vi "Suggestion Box Panel.vi"(11 "Suggestion Box":refnum<class "Suggestion Box.lvclass">) -> ()   [LabVIEW 2016, in "Suggestion Box.lvclass"]
doc: "Suggestion Box panel process.\n--------------------\nCopyright (c) 2019 Analog Devices, Inc. All rights reserved.\n\nRedistribution and use in source and binary forms, with or without modification,\nare permitted provided that the following conditions are met:\n - Redistributions of source code must retain the above copyright notice, this\n list of conditions and the following disclaimer.\n - Redistributions in binary form must reproduce the above copyright notice,\n this list of conditions and the following disclaimer in the documentation\n and/or other materials provided with the distribution.\n - Modified versions of the software must be conspicuously marked as such.\n - This software is licensed solely and exclusively for use with\n processors/products manufactured by or for Analog Devices, Inc.\n - This software may not be combined or merged with other code in any manner\n that would cause the software to become subject to terms and conditions\n which differ from those listed here.\n - Neither the name of Analog Devices, Inc. nor the names of its contributors\n may be used to endorse or promote products derived from this software\n without specific prior written permission.\n - The use of this software may or may not infringe the patent rights of one or\n more patent holders. This license does not release you from the requirement\n that you obtain separate licenses from these patent holders to use this\n software.\n\nTHIS SOFTWARE IS PROVIDED BY ANALOG DEVICES, INC. AND CONTRIBUTORS \"AS IS\" AND\nANY EXPRESS OR IMPLIED WARRANTIES, INCLUDING, BUT NOT LIMITED TO,\nNON-INFRINGEMENT, TITLE, MERCHANTABILITY AND FITNESS FOR A PARTICULAR PURPOSE\nARE DISCLAIMED. IN NO EVENT SHALL ANALOG DEVICES, INC. OR CONTRIBUTORS BE LIABLE\nFOR ANY DIRECT, INDIRECT, INCIDENTAL, SPECIAL, EXEMPLARY, PUNITIVE OR\nCONSEQUENTIAL DAMAGES (INCLUDING, BUT NOT LIMITED TO, DAMAGES ARISING OUT OF\nCLAIMS OF INTELLECTUAL PROPERTY RIGHTS INFRINGEMENT; PROCUREMENT OF SUBSTITUTE\nGOODS OR SERVICES; LOSS OF USE, DATA, OR PROFITS; OR BUSINESS INTERRUPTION)\nHOWEVER CAUSED AND ON ANY THEORY OF LIABILITY, WHETHER IN CONTRACT, STRICT\nLIABILITY, OR TORT (INCLUDING NEGLIGENCE OR OTHERWISE) ARISING IN ANY WAY OUT OF\nTHE USE OF THIS SOFTWARE, EVEN IF ADVISED OF THE POSSIBILITY OF SUCH DAMAGE.\n\n2019-01-10-7CBSD SLA"
uses:
  Suggestion Box.lvclass
  Suggestion Box.lvclass/Suggestion Box.ctl
  Events/Update Data.ctl
  <vilib>/Utility/miscctls.llb/LVPositionTypeDef.ctl
  Autocomplete/String Match.ctl
  Autocomplete/Segment.ctl
  <vilib>/Utility/miscctls.llb/LVFontTypeDef.ctl
panel:
  out "Cover":picture
  out "Text":string
  out "List":i32(listbox)=-1
  # "Copyright (c) 2019 Analog Devices, Inc.  All rights reserved.\n\nRedistribution and use in source and binary forms, with or without modification,\nare permitted provided that the following conditions are met:\n  - Redistributions of source code must retain the above copyright notice, this\n    list of conditions and the following disclaimer.\n  - Redistributions in binary form must reproduce the above copyright notice,\n    this list of conditions and the following disclaimer in the documentation\n    and/or other materials provided with the distribution.\n  - Modified versions of the software must be conspicuously marked as such.\n  - This software is licensed solely and exclusively for use with\n    processors/products manufactured by or for Analog Devices, Inc.\n  - This software may not be combined or merged with other code in any manner\n    that would cause the software to become subject to terms and conditions\n    which differ from those listed here.\n  - Neither the name of Analog Devices, Inc. nor the names of its contributors\n    may be used to endorse or promote products derived from this software\n    without specific prior written permission.\n  - The use of this software may or may not infringe the patent rights of one or\n    more patent holders.  This license does not release you from the requirement\n    that you obtain separate licenses from these patent holders to use this\n    software.\n\nTHIS SOFTWARE IS PROVIDED BY ANALOG DEVICES, INC. AND CONTRIBUTORS \"AS IS\" AND\nANY EXPRESS OR IMPLIED WARRANTIES, INCLUDING, BUT NOT LIMITED TO,\nNON-INFRINGEMENT, TITLE, MERCHANTABILITY AND FITNESS FOR A PARTICULAR PURPOSE\nARE DISCLAIMED. IN NO EVENT SHALL ANALOG DEVICES, INC. OR CONTRIBUTORS BE LIABLE\nFOR ANY DIRECT, INDIRECT, INCIDENTAL, SPECIAL, EXEMPLARY, PUNITIVE OR\nCONSEQUENTIAL DAMAGES (INCLUDING, BUT NOT LIMITED TO, DAMAGES ARISING OUT OF\nCLAIMS OF INTELLECTUAL PROPERTY RIGHTS INFRINGEMENT; PROCUREMENT OF SUBSTITUTE\nGOODS OR SERVICES; LOSS OF USE, DATA, OR PROFITS; OR BUSINESS INTERRUPTION)\nHOWEVER CAUSED AND ON ANY THEORY OF LIABILITY, WHETHER IN CONTRACT, STRICT\nLIABILITY, OR TORT (INCLUDING NEGLIGENCE OR OTHERWISE) ARISING IN ANY WAY OUT OF\nTHE USE OF THIS SOFTWARE, EVEN IF ADVISED OF THE POSSIBILITY OF SUCH DAMAGE.\n\n2019-01-10-7CBSD SLA"
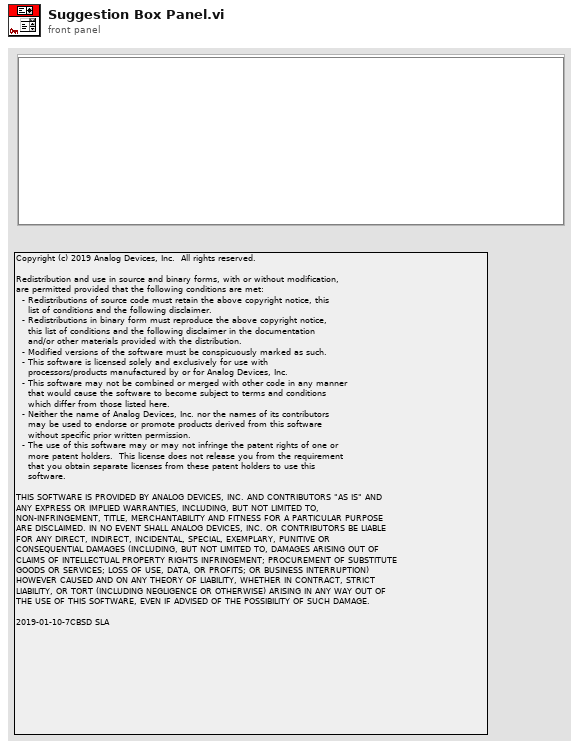
[diagram p1: front panel]
types:
  T1 = enum32{"Invalid", "Standard", "Closed", "Hidden", "Minimized", "Maximized"}
  T2 = enum32{"invalid app kind", "Development System", "Run Time System", "Student Edition", "Embedded LabVIEW", "Evaluation", "Custom"}
  T3 = typedef "LVPoint32TypeDef.ctl" = cluster{"Horizontal":i32, "Vertical":i32}
  T4 = typedef "LVRectTypeDef.ctl" = cluster{"Left":i16, "Top":i16, "Right":i16, "Bottom":i16}
  T5 = typedef "eventvkey.ctl" = enum16{"ASCII", "Enter", "Return", "Shift", "Ctrl", "Alt", "Cmd", "Opt", "Caps", "NumLock", "Clear", "Break", "Up", "Down", "Left", "Right", "Insert", "Delete", "Home", "End", "PageUp", "PageDown", "Escape", "Help", "Pause", "ScrollLock", "F1", "F2", "F3", "F4", "F5", "F6", "F7", "F8", "F9", "F10", "F11", "F12", "F13", "F14", "F15", "F16", "F17", "F18", "F19", "F20", "F21", "F22", "F23", "F24", "Play", "VolumeUp", "VolumeDown", "Mute", "Two Byte Char"}
  T6 = typedef "LVPositionTypeDef.ctl" = cluster{"Left":i32, "Top":i32}
  T7 = typedef "Suggestion Box.lvclass/String Match.ctl" = cluster{"Source":string, "Segments":T8[], "Match Start":i32, "Edit Distance":i32}
  T8 = typedef "Suggestion Box.lvclass/Segment.ctl" = cluster{"Start":i32, "End":i32, "Match?":bool}
  T9 = typedef "Suggestion Box.lvclass/Update Data.ctl" = cluster{"Query":string, "Keywords":string[], "Position":T6}
  T10 = typedef "LVFontTypeDef.ctl" = cluster{"Font Name":string, "Size":u16, "Bold":bool, "Italic":bool, "Underline":bool, "Strikeout":bool, "Color":u32}
  T11 = cluster{"Core":cluster{"Current VI Reference":refnum<vi>, "Close Panel on Exit?":bool}, "Text":refnum<vi>, "List":refnum<vi>, "Cover":refnum<vi>, "Update Data":T9, "Suggestions":T7[], "Font":T10, "T":i32}
  T12 = typedef "Rendezvous RefNum" = refnum<k1>
  T13 = cluster{"Current VI Reference":refnum<vi>, "Close Panel on Exit?":bool}
  T14 = typedef "Suggestion Box.lvclass/User Events.ctl" = cluster{"Exit":refnum<user-event>, "Update":refnum<user-event>, "Resolve":refnum<user-event>, "Navigate":refnum<user-event>, "Font":refnum<user-event>}
  T15 = typedef "LVBoundsTypeDef.ctl" = cluster{"Width":u32, "Height":u32}
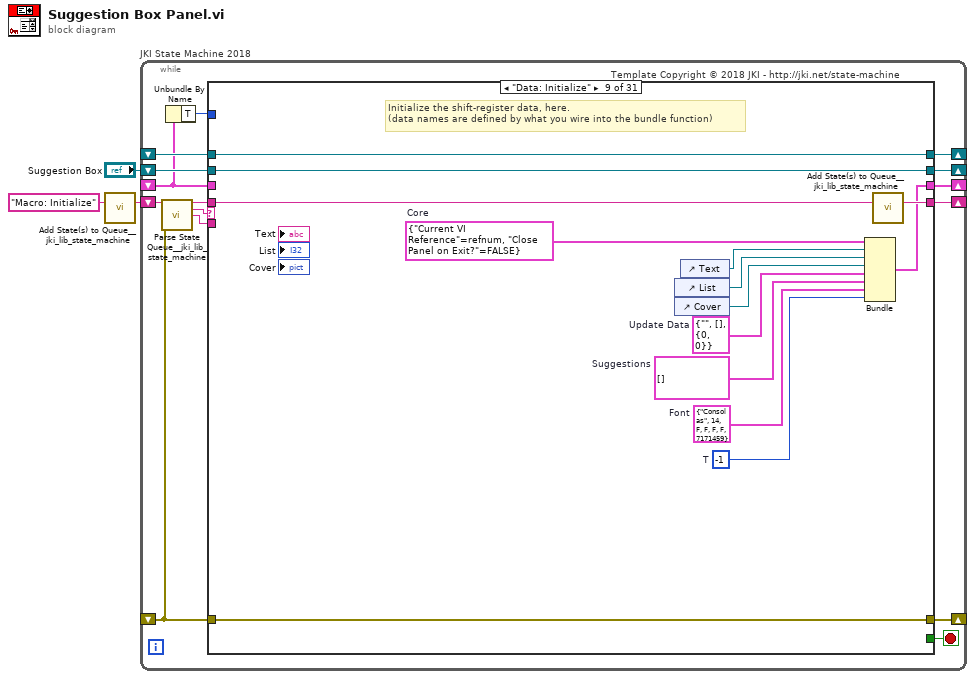
[diagram p0: block diagram]
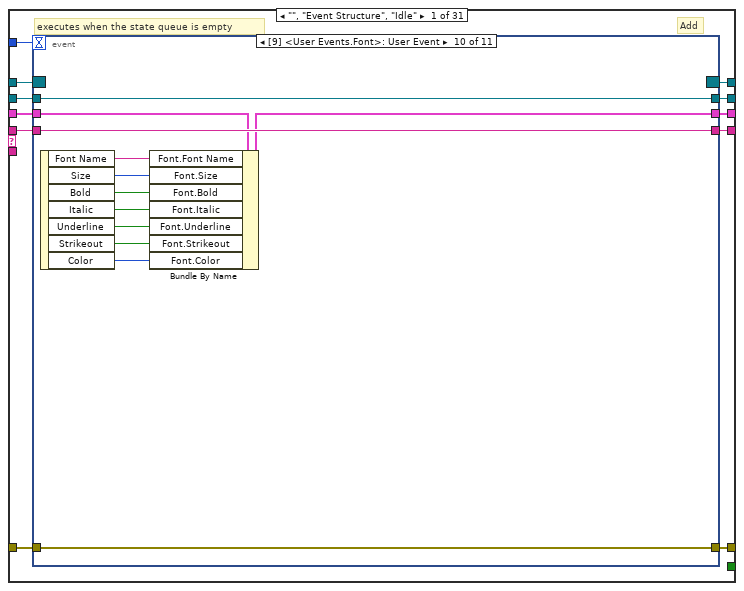
[diagram p2: hidden frame]
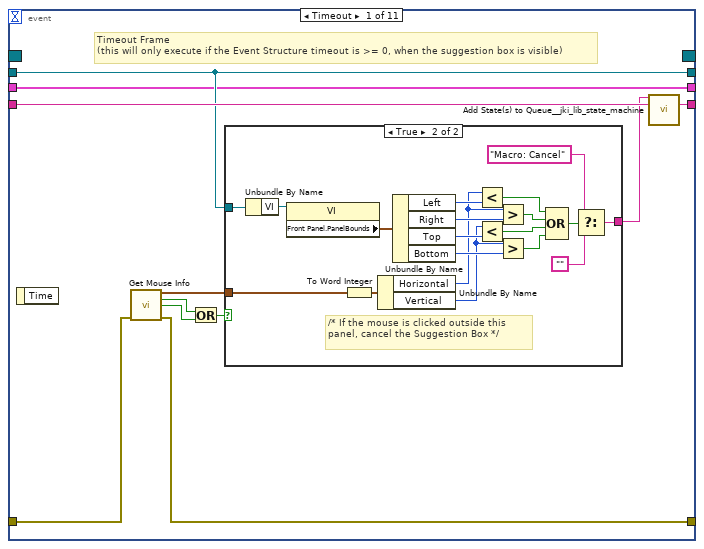
[diagram p3: hidden frame]
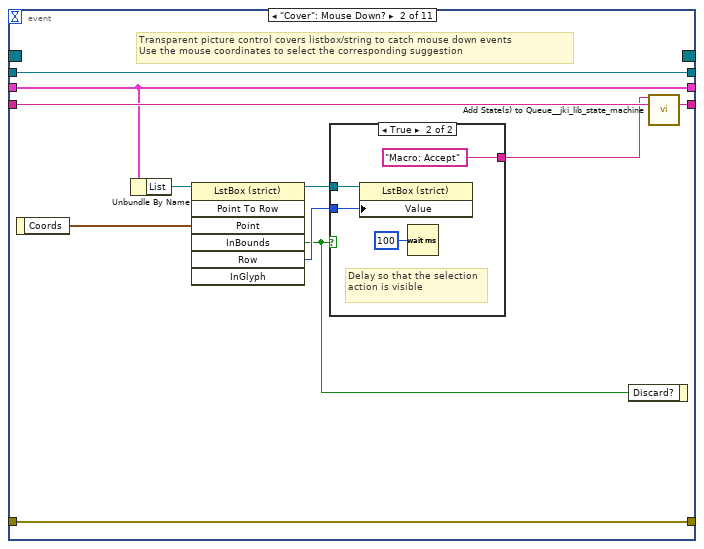
[diagram p5: hidden frame]
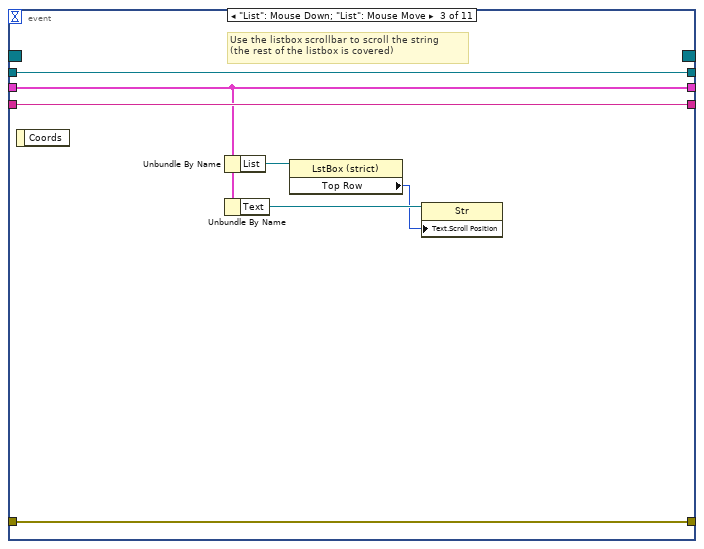
[diagram p7: hidden frame]
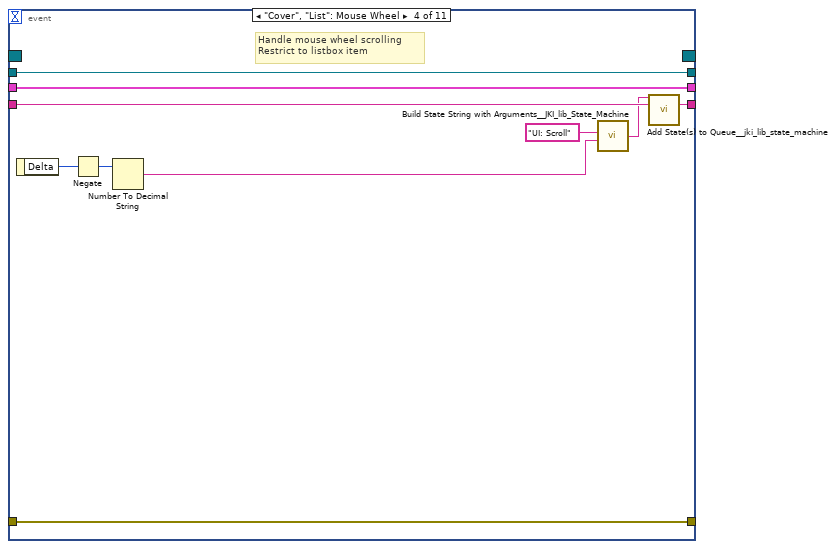
[diagram p8: hidden frame]
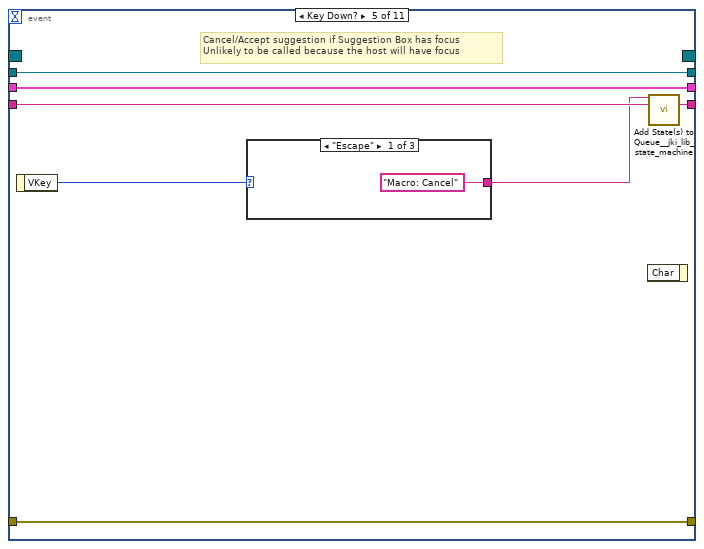
[diagram p9: hidden frame]
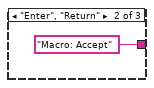
[diagram p10: hidden frame]
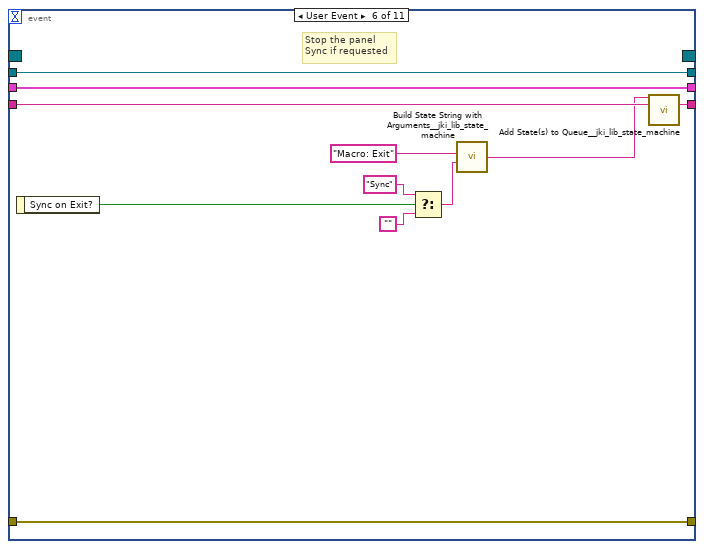
[diagram p12: hidden frame]
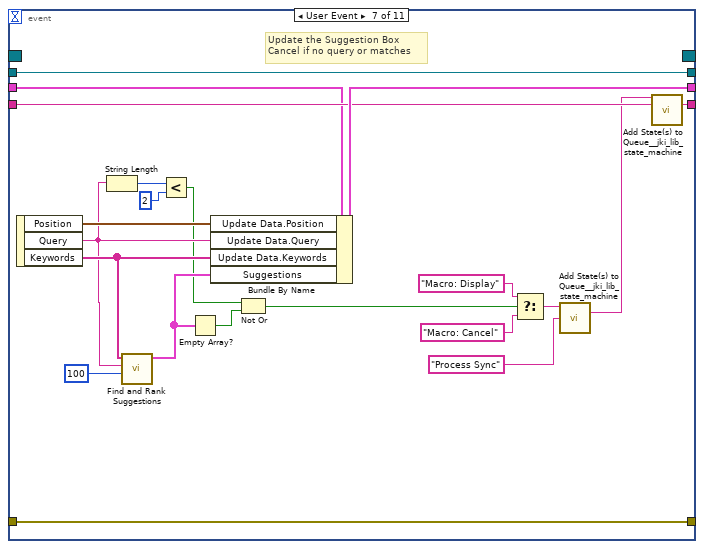
[diagram p13: hidden frame]
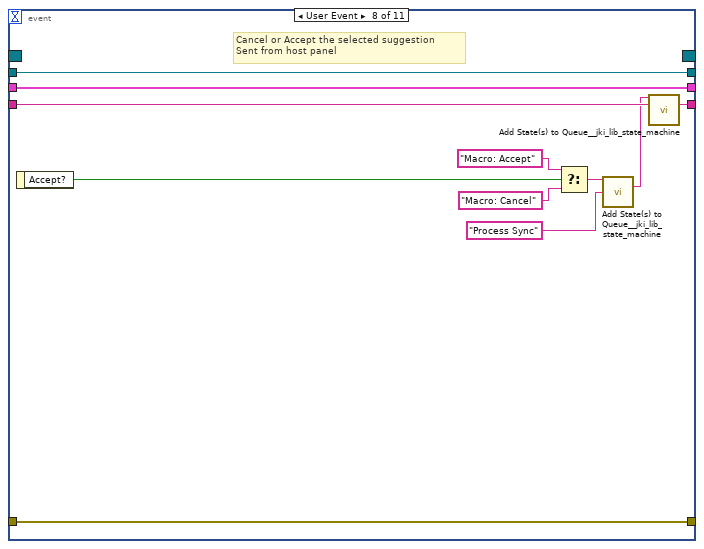
[diagram p14: hidden frame]
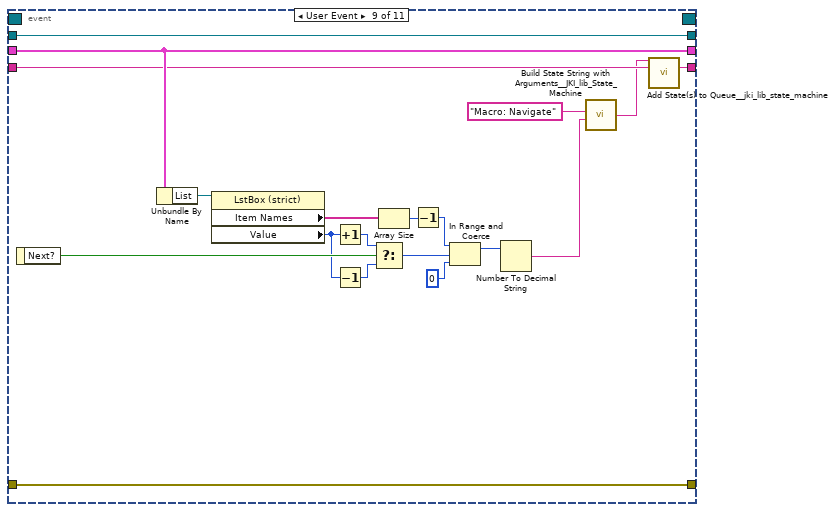
[diagram p15: hidden frame]
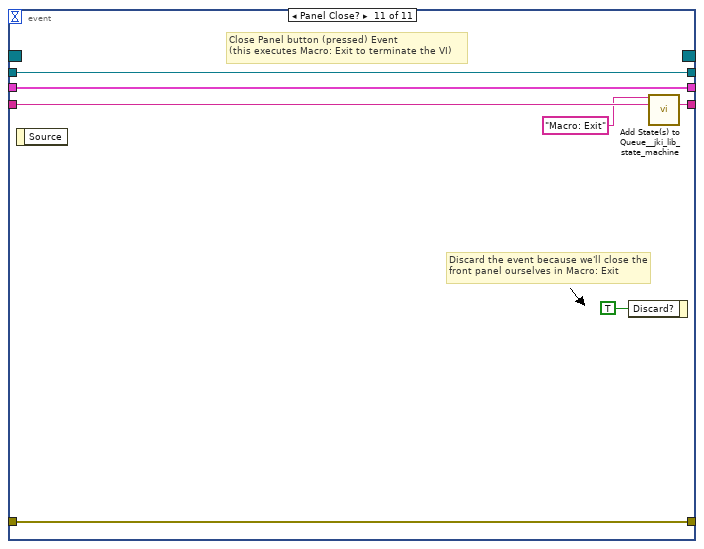
[diagram p16: hidden frame]
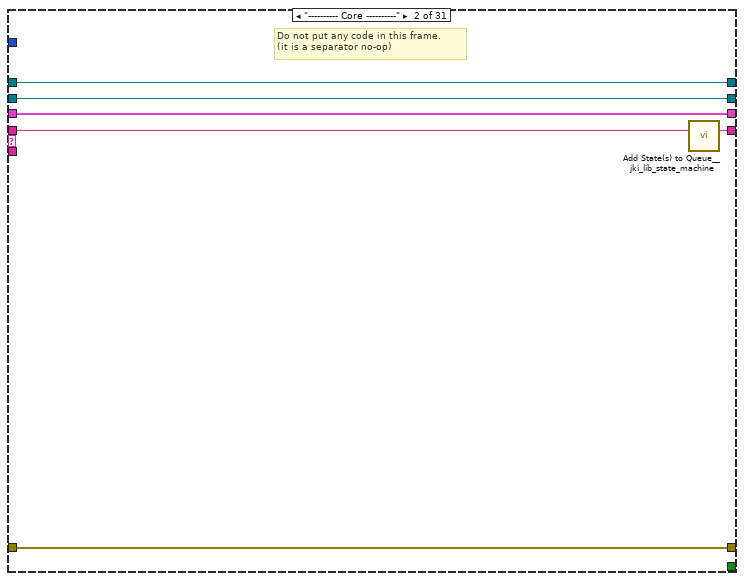
[diagram p17: hidden frame]
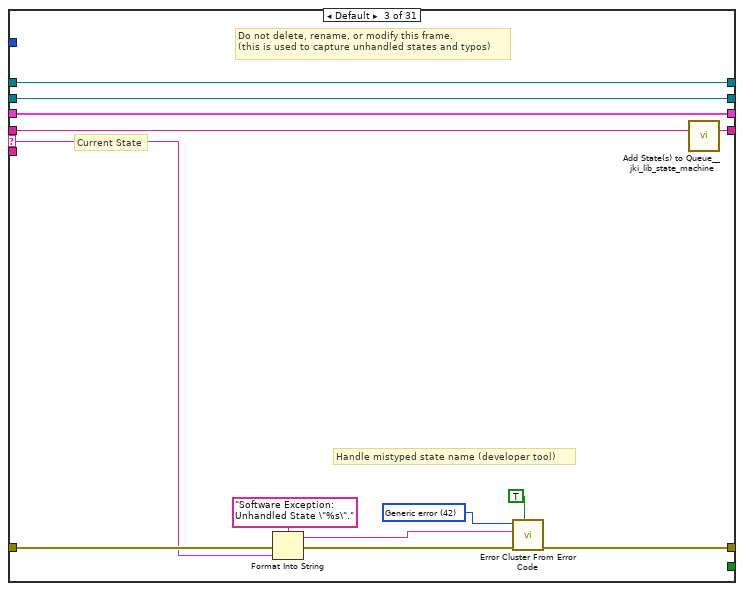
[diagram p18: hidden frame]
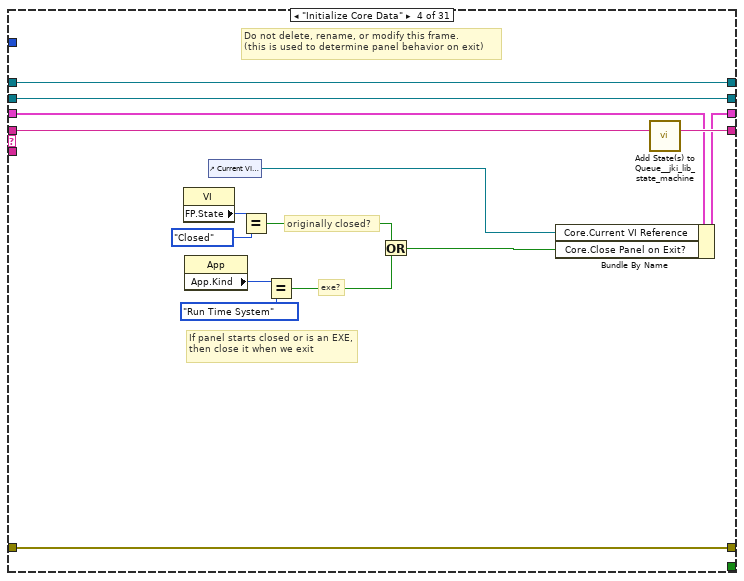
[diagram p19: hidden frame]
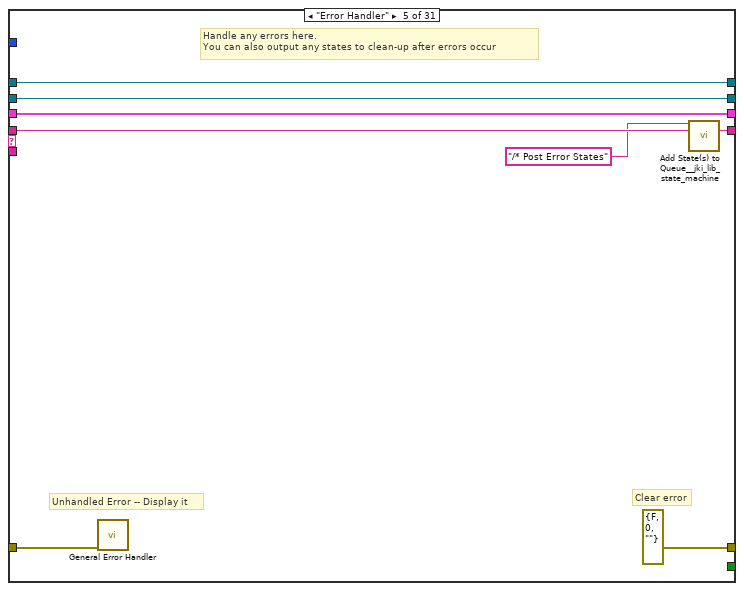
[diagram p20: hidden frame]
diagram:
  n1 = call <vilib>:"Add State(s) to Queue__jki_lib_state_machine.vi"("State(s) in (\"\")"="Macro: Initialize") -> ("States Out"=w3:string)  [unwired: 14 in]
  n2 = while "JKI State Machine 2018" {
    shift-right: [w11] -> _
    shift-left: _ -> [w4]
    shift-right: [w14] -> _
    shift-left: _ -> [w10]
    shift-right: [w13] -> _
    shift-left: w3 -> [w15]
    shift-right: [w8] -> _
    shift-left: "Suggestion Box" -> [w9]
    shift-right: [w7] -> _
    shift-left: _ -> [w6]
    stop <- w12 stop-if-true
    # "Template Copyright © 2018 JKI - http://jki.net/state-machine"
    n3 = call <vilib>:"Parse State Queue__jki_lib_state_machine.vi"("State Queue"=w15, "Error In (no error)"=w10) -> ("Remaining States"=w17:string, "Current State"=w18:string, "Arguments"=w16:string)  [unwired: 11 in]
    n4 = Unbundle By Name(w4) -> ("T"=w5:i32)
    n5 = case shown="\"Data: Initialize\"" w18 {
      selector: w18 -> [_ _ w190 _ _ _ _ _ _ _ _ _ _ _ _ _ _ _ _ _ _ _ _ _ _ _ _ _ _ _ _]
      tunnel: w17 -> [w29 w187 w194 w215 w223 w232 w239 w245 w259 w267 w279 w290 w299 w308 w314 w334 w342 w355 w434 w448 w487 w505 w532 w543 w549 w556 w563 w575 w582 w589 w602]
      tunnel: w16 -> [_ _ _ _ _ _ _ _ _ _ _ _ w291 _ _ _ w337 w349 w430 _ _ w490 w514 _ _ _ _ w568 _ _ w593]
      tunnel: w4 -> [w27 w184 w192 w208 w220 w230 w237 w242 _ w265 w271 w288 w296 w301 w311 w319 w340 w351 w429 w442 w462 w492 w515 w540 w546 w553 w560 w572 w579 w586 w592]
      tunnel: [w26 w185 w196 w212 errorcluster {"status"=FALSE, "code"=0, "source"=""} ("error out") w225 w236 w243 w248 w262 w268 w283 w297 w302 w312 w332 w338 w352 w424 w446 w485 w503 w530 w541 w547 w554 w561 w573 w580 w587 w600] -> w14
      tunnel: w10 -> [w25 w185 w195 w212 w219 w226 w236 w243 w248 w263 w269 w284 w297 w300 w312 w332 w339 w353 w423 w446 w485 w503 w530 w541 w547 w554 w561 w573 w580 w587 w600]
      tunnel: [w28 w186 w193 w214 w222 w231 w238 w244 w258 w266 w278 w289 w298 w307 w313 w333 w341 w354 w433 w447 w486 w504 w531 w542 w548 w555 w562 w574 w581 w588 w601] -> w13
      tunnel: [_ _ _ _ _ _ TRUE _ _ _ _ _ _ _ _ _ _ _ _ _ _ _ _ _ _ _ _ _ _ _ _] -> w12
      tunnel: [w24 w184 w192 w213 w220 w230 w237 w242 w257 w265 w271 w281 w293 w301 w311 w319 w340 w351 w429 w438 w462 w492 w515 w540 w546 w553 w560 w572 w579 w586 w592] -> w11
      tunnel: w5 -> [w23 _ _ _ _ _ _ _ _ _ _ _ _ _ _ _ _ _ _ _ _ _ _ _ _ _ _ _ _ _ _]
      tunnel: w9 -> [w22 w183 w189 w202 w217 w227 w234 w241 w255 w261 w273 w286 w295 w305 w310 w328 w336 w348 w432 w445 w476 w502 w529 w536 w545 w551 w559 w571 w578 w585 w599]
      tunnel: [w21 w183 w189 w202 w217 w227 w234 w241 w255 w261 w272 w285 w295 w305 w310 w328 w336 w348 w432 w445 w476 w502 w529 w536 w545 w551 w559 w571 w578 w585 w599] -> w8
      tunnel: [w19 w182 w188 w201 w216 w224 w233 w240 w254 w264 w277 w287 w294 w303 w309 w327 w335 w347 w431 w444 w475 w501 w528 w535 w544 w550 w558 w570 w577 w584 w598] -> w7
      tunnel: w6 -> [w20 w182 w188 w201 w216 w224 w233 w240 w254 _ w277 w287 w294 w303 w309 w327 w335 w347 w431 w444 w475 w501 w528 w535 w544 w550 w558 w570 w577 w584 w598]
      frame "", "Event Structure", "Idle" {
        # "Add"
        # "executes when the state queue is empty"
        n6 = event shown="[9] <User Events.Font>: User Event" {
          selector: w20 -> [_ _ _ _ _ _ _ _ _ _ _]
          dyn-events: [_ _ _ _ _ _ _ _ _ _ _] -> w19
          timeout: w23 -> [_ _ _ _ _ _ _ _ _ _ _]
          tunnel: w29 -> [w40 w65 w81 w86 w93 w111 w128 w139 w154 w174 w181]
          tunnel: [w39 w66 w81 w87 w94 w110 w129 w140 w155 w174 w180] -> w28
          tunnel: w27 -> [w32 w60 w76 w89 w97 w108 w117 w142 w160 w172 w178]
          tunnel: [w34 w70 w80 w91 w98 w109 w132 w143 w162 w173 w179] -> w26
          tunnel: w25 -> [w33 w70 w80 w91 w98 w109 w132 w143 w162 w173 w179]
          tunnel: [w32 w60 w76 w89 w97 w108 w130 w142 w160 w170 w178] -> w24
          tunnel: w22 -> [w38 w63 w79 w90 w96 w107 w131 w141 w161 w171 w175]
          tunnel: [w38 w63 w79 w90 w96 w107 w131 w141 w161 w171 w175] -> w21
          event Timeout {
            # "Timeout Frame\n(this will only execute if the Event Structure timeout is >= 0, when the suggestion box is visible)"
            n7 = event-data() -> ()  [unwired: 1 in, 1 out]
            n8 = call "Get Mouse Info.vi"("error in (no error)"=w33) -> ("Coordinates"=w35:T3, "Left Mouse Button?"=w30:bool, "Right Mouse Button?"=w31:bool, "error out"=w34:errorcluster)  [unwired: 11 in]
            n9 = Or(x=w30, y=w31) -> (x .or. y?=w36:bool)
            n10 = case shown="True" w36 {
              tunnel: w38 -> [_ w59]
              tunnel: [_ w58] -> w37
              tunnel: w35 -> [_ w42]
              frame False {
              }
              frame True {
                # "/* If the mouse is clicked outside this panel, cancel the Suggestion Box */"
                n11 = Unbundle By Name(w59) -> ("VI"=w57:refnum<vi>)
                n12 = property class="VI"(reference=w57) -> ("Front Panel.PanelBounds"=w56:T4)  [unwired: 1 in, 2 out]
                n13 = To Word Integer(number=w42) -> (16bit integer=w41:cluster{"Horizontal":i16, "Vertical":i16})
                n14 = Unbundle By Name(w41) -> ("Horizontal"=w44:i16, "Vertical"=w43:i16)
                n15 = Unbundle By Name(w56) -> ("Left"=w54:i16, "Right"=w55:i16, "Top"=w53:i16, "Bottom"=w52:i16)
                n16 = Less?(x=w44, y=w54) -> (x < y?=w51:bool)
                n17 = Less?(x=w43, y=w53) -> (x < y?=w49:bool)
                n18 = Greater?(x=w44, y=w55) -> (0:w50:bool)
                n19 = Greater?(x=w43, y=w52) -> (0:w48:bool)
                n20 = Compound Arithmetic op=OR(w51, w50, w49, w48) -> (w45:bool)
                n21 = Select(t="Macro: Cancel", s=w45, f="") -> (s? t:f=w58:string)
              }
            }
            n22 = call <vilib>:"Add State(s) to Queue__jki_lib_state_machine.vi"("State(s) in Front (\"\")"=w37, "State(s) in (\"\")"=w40) -> ("States Out"=w39:string)  [unwired: 13 in]
          }
          event "Cover": Mouse Down? {
            # "Transparent picture control covers listbox/string to catch mouse down events\nUse the mouse coordinates to select the corresponding suggestion"
            n23 = event-data() -> ("Coords"=w62:T3)  [unwired: 1 in]
            n24 = Unbundle By Name(w60) -> ("List"=w61:refnum<vi>)
            n25 = invoke class="LstBox (strict)" method="Point To Row"(reference=w61, "Point"=w62) -> (reference out=w69:refnum<vi>, "InBounds"=w67:bool, "Row"=w68:i32)  [unwired: 5 in, 4 out]
            n26 = case shown="True" w67 {
              tunnel: w69 -> [_ w74]
              tunnel: w68 -> [_ w71]
              tunnel: [_ "Macro: Accept"] -> w64
              frame False {
              }
              frame True {
                # "Delay so that the selection action is visible"
                n27 = property class="LstBox (strict)"(reference=w74, "Value"=w71) -> ()  [unwired: 1 in, 2 out]
                n28 = Wait (ms)(milliseconds to wait=u32 100) -> ()  [unwired: 1 out]
              }
            }
            n29 = event-data("Discard?"=w67) -> ()  [unwired: 1 in, 1 out]
            n30 = call <vilib>:"Add State(s) to Queue__jki_lib_state_machine.vi"("State(s) in Front (\"\")"=w64, "State(s) in (\"\")"=w65) -> ("States Out"=w66:string)  [unwired: 13 in]
          }
          event "List": Mouse Down; "List": Mouse Move {
            # "Use the listbox scrollbar to scroll the string\n(the rest of the listbox is covered)"
            n31 = event-data() -> ()  [unwired: 1 in, 1 out]
            n32 = Unbundle By Name(w76) -> ("List"=w75:refnum<vi>)
            n33 = Unbundle By Name(w76) -> ("Text"=w78:refnum<vi>)
            n34 = property class="LstBox (strict)"(reference=w75) -> ("Top Row"=w77:i32)  [unwired: 1 in, 2 out]
            n35 = property class="Str"(reference=w78, "Text.Scroll Position"=w77) -> ()  [unwired: 1 in, 2 out]
          }
          event "Cover", "List": Mouse Wheel {
            # "Handle mouse wheel scrolling\nRestrict to listbox item"
            n36 = event-data() -> ("Delta"=w88:i32)  [unwired: 1 in]
            n37 = Negate(x=w88) -> (-x=w84:i32)
            n38 = Number To Decimal String(number=w84) -> (decimal integer string=w83:string)  [unwired: 1 in]
            n39 = call <vilib>:"Build State String with Arguments__JKI_lib_State_Machine.vi"("Arguments (\"\")"=w83, "State"="UI: Scroll") -> ("State with Arguments"=w82:string)  [unwired: 4 in]
            n40 = call <vilib>:"Add State(s) to Queue__jki_lib_state_machine.vi"("State(s) in Front (\"\")"=w82, "State(s) in (\"\")"=w86) -> ("States Out"=w87:string)  [unwired: 13 in]
          }
          event Key Down? {
            # "Cancel/Accept suggestion if Suggestion Box has focus\nUnlikely to be called because the host will have focus"
            n41 = event-data() -> ("VKey"=w95:T5)  [unwired: 1 in]
            n42 = case shown="\"Escape\"" w95 {
              tunnel: ["Macro: Cancel" "Macro: Accept" _] -> w92
              frame "Escape" {
              }
              frame "Enter", "Return" {
              }
              frame Default {
              }
            }
            n43 = event-data() -> ()  [unwired: 2 in, 1 out]
            n44 = call <vilib>:"Add State(s) to Queue__jki_lib_state_machine.vi"("State(s) in Front (\"\")"=w92, "State(s) in (\"\")"=w93) -> ("States Out"=w94:string)  [unwired: 13 in]
          }
          event User Event {
            # "Stop the panel\nSync if requested"
            n45 = event-data() -> ("Sync on Exit?"=w102:bool)  [unwired: 1 in]
            n46 = Select(t="Sync", s=w102, f="") -> (s? t:f=w104:string)
            n47 = call <vilib>:"Build State String with Arguments__jki_lib_state_machine.vi"("Arguments (\"\")"=w104, "State"="Macro: Exit") -> ("State with Arguments"=w101:string)  [unwired: 4 in]
            n48 = call <vilib>:"Add State(s) to Queue__jki_lib_state_machine.vi"("State(s) in Front (\"\")"=w101, "State(s) in (\"\")"=w111) -> ("States Out"=w110:string)  [unwired: 13 in]
          }
          event User Event {
            # "Update the Suggestion Box\nCancel if no query or matches"
            n49 = event-data() -> ("Position"=w123:T6, "Query"=w115:string, "Keywords"=w116:string[])  [unwired: 1 in]
            n50 = String Length(string=w115) -> (length=w114:i32)
            n51 = call "Find and Rank Suggestions.vi"("Suggestion Limit (-1: No limit)"=100, "Query"=w115, "Keywords"=w116) -> ("Suggestions"=w118:T7[])  [unwired: 7 in, 1 out]
            n52 = Less?(x=w114, y=2) -> (x < y?=w112:bool)
            n53 = Empty Array?(array=w118) -> (empty?=w127:bool)
            n54 = Bundle By Name(cluster=w117, "Update Data.Position"=w123, "Update Data.Query"=w115, "Update Data.Keywords"=w116, "Suggestions"=w118) -> (w130:T11)
            n55 = Not Or(1:w127, 2:w112) -> (0:w124:bool)
            n56 = Select(t="Macro: Display", s=w124, f="Macro: Cancel") -> (s? t:f=w122:string)
            n57 = call <vilib>:"Add State(s) to Queue__jki_lib_state_machine.vi"("State(s) in Front (\"\")"=w122, "State(s) at Back (\"\")"="Process Sync") -> ("States Out"=w120:string)  [unwired: 13 in]
            n58 = call <vilib>:"Add State(s) to Queue__jki_lib_state_machine.vi"("State(s) in Front (\"\")"=w120, "State(s) in (\"\")"=w128) -> ("States Out"=w129:string)  [unwired: 13 in]
          }
          event User Event {
            # "Cancel or Accept the selected suggestion\nSent from host panel"
            n59 = event-data() -> ("Accept?"=w134:bool)  [unwired: 1 in]
            n60 = Select(t="Macro: Accept", s=w134, f="Macro: Cancel") -> (s? t:f=w138:string)
            n61 = call <vilib>:"Add State(s) to Queue__jki_lib_state_machine.vi"("State(s) in Front (\"\")"=w138, "State(s) at Back (\"\")"="Process Sync") -> ("States Out"=w133:string)  [unwired: 13 in]
            n62 = call <vilib>:"Add State(s) to Queue__jki_lib_state_machine.vi"("State(s) in Front (\"\")"=w133, "State(s) in (\"\")"=w139) -> ("States Out"=w140:string)  [unwired: 13 in]
          }
          event User Event {
            n63 = event-data() -> ("Next?"=w156:bool)  [unwired: 1 in]
            n64 = Unbundle By Name(w160) -> ("List"=w159:refnum<vi>)
            n65 = property class="LstBox (strict)"(reference=w159) -> ("Item Names"=w150:string[], "Value"=w151:i32)  [unwired: 1 in, 2 out]
            n66 = Increment(x=w151) -> (x+1=w158:i32)
            n67 = Decrement(x=w151) -> (x-1=w157:i32)
            n68 = Select(t=w158, s=w156, f=w157) -> (s? t:f=w153:i32)
            n69 = Array Size(array=w150) -> (size(s)=w149:i32)
            n70 = Decrement(x=w149) -> (x-1=w144:i32)
            n71 = In Range and Coerce(upper limit=w144, x=w153, lower limit=0) -> (coerced(x)=w148:i32)  [unwired: 1 out]
            n72 = Number To Decimal String(number=w148) -> (decimal integer string=w147:string)  [unwired: 1 in]
            n73 = call <vilib>:"Build State String with Arguments__JKI_lib_State_Machine.vi"("Arguments (\"\")"=w147, "State"="Macro: Navigate") -> ("State with Arguments"=w145:string)  [unwired: 4 in]
            n74 = call <vilib>:"Add State(s) to Queue__jki_lib_state_machine.vi"("State(s) in Front (\"\")"=w145, "State(s) in (\"\")"=w154) -> ("States Out"=w155:string)  [unwired: 13 in]
          }
          event User Event {
            n75 = event-data() -> ("Font Name"=w163:string, "Size"=w164:u16, "Bold"=w165:bool, "Italic"=w166:bool, "Underline"=w167:bool, "Strikeout"=w168:bool, "Color"=w169:u32)  [unwired: 1 in]
            n76 = Bundle By Name(cluster=w172, "Font.Font Name"=w163, "Font.Size"=w164, "Font.Bold"=w165, "Font.Italic"=w166, "Font.Underline"=w167, "Font.Strikeout"=w168, "Font.Color"=w169) -> (w170:T11)
          }
          event Panel Close? {
            # "Discard the event because we'll close the front panel ourselves in Macro: Exit"
            # "Close Panel button (pressed) Event\n(this executes Macro: Exit to terminate the VI)"
            n77 = event-data() -> ()  [unwired: 1 in, 1 out]
            n78 = event-data("Discard?"=TRUE) -> ()  [unwired: 1 in, 1 out]
            n79 = call <vilib>:"Add State(s) to Queue__jki_lib_state_machine.vi"("State(s) in Front (\"\")"="Macro: Exit", "State(s) in (\"\")"=w181) -> ("States Out"=w180:string)  [unwired: 13 in]
          }
        }
      }
      frame "---------- Core ----------" {
        # "Do not put any code in this frame.\n(it is a separator no-op)"
        n80 = call <vilib>:"Add State(s) to Queue__jki_lib_state_machine.vi"("State(s) in (\"\")"=w187) -> ("States Out"=w186:string)  [unwired: 14 in]
      }
      frame Default {
        w199 = 42 items=["No error", "Argument error", "Memory is full", "Out of zone", "End of file", "File already open", "Generic file I/O error", "File not found", "File permission error", "Disk is full", "Duplicate path", "Too many files open", "System feature not enabled", "Resource file not found", "Cannot add resource", "Resource not found", "Image not found", "Image memory error", "Pen does not exist", "Config type invalid", "Config token not found", "Config parse error", "Config memory error", "Bad external code format", "Bad external code offset", "External code not present", "Null window", "Destroy window error", "Null menu", "Print aborted", "Bad print record", "Print driver error", "Windows error during printing", "Memory error during printing", "Print dialog error", "Generic print error", "Invalid device refnum", "Device not found", "Device parameter error", "Device unit error", "Cannot open device", "Device call aborted", "Generic error", "Cancelled by user", "Object ID too low", "Object ID too high", "Object not in heap", "Unknown heap", "Unknown object (invalid DefProc)", "Unknown object (DefProc not in table)", "Message out of range", "Invalid (null) method", "Unknown message", "Manager call not supported", "Bad address", "Network operation in progress", "Network operation timed out", "Connection is busy", "Network attribute not supported", "Network error", "Address in use", "System out of memory", "Connection aborted", "Connection refused", "Not connected", "Already connected", "Connection closed", "Initialization error (interapplication manager)", "Bad occurrence", "Wait on unbound occurrence handler", "Occurrence queue overflow", "Datalog type conflict", "Unused", "Unrecognized type (interapplication manager)", "Memory corrupt", "Failed to make temporary DLL", "Old CIN version", "Drag socket not found", "Failed to load drop-object", "Failed to register OLE object", "Failed to release OLE object", "Format specifier type mismatch", "Unknown format specifier", "Too few format specifiers", "Too many format specifiers", "Scan failed", "Newer CIN version", "Error converting to variant", "Runtime menu error", "Password tampered", "Variant attribute not found", "Incompatible variant data type", "Event data is not available", "Event Store is not present", "Occurrence is not found", "Event Queue is not created", "Event info is not available", "Refnum passed is NULL", "Error retrieving Class GUID", "Error retrieving CoClass GUID", "Error retrieving TypeLib GUID.", "Bad built application magic bytes.", "Specific driver is different from the specific driver associated with the Logical Name.", "There is no session opened to the class driver.", "Max Error", "MAX - Error with config objects", "MAX - Error loading configuration", "MAX - Group not supported"]
        # "Current State"
        # "Do not delete, rename, or modify this frame.\n(this is used to capture unhandled states and typos)"
        # "Handle mistyped state name (developer tool)"
        n81 = Format Into String(format string="Software Exception: Unhandled State \"%s\"." ("message"), error in=w195, w190) -> (resulting string=w198:string, error out=w197:errorcluster)  [unwired: 1 in]
        n82 = call <vilib>:"Error Cluster From Error Code.vi"("show call chain? (False)"=TRUE, "error in (no error)"=w197, "error message (\"\")"=w198, "error code (0)"=w199) -> ("error out"=w196:errorcluster)  [unwired: 5 in]
        n83 = call <vilib>:"Add State(s) to Queue__jki_lib_state_machine.vi"("State(s) in (\"\")"=w194) -> ("States Out"=w193:string)  [unwired: 14 in]
      }
      frame "Initialize Core Data" {
        # "Do not delete, rename, or modify this frame.\n(this is used to determine panel behavior on exit)"
        # "originally closed?"
        # "exe?"
        # "If panel starts closed or is an EXE, then close it when we exit"
        n84 = property class="VI"() -> ("FP.State"=w205:T1)  [unwired: 2 in, 2 out]
        n85 = property class="App"() -> ("App.Kind"=w211:T2)  [unwired: 2 in, 2 out]
        n86 = control-ref of="Current VI Reference"() -> (w206:refnum<vi>)
        n87 = Equal?(x=w205, y=T1."Closed" ("Front Panel Window:State")) -> (x = y?=w203:bool)
        n88 = Equal?(x=w211, y=T2."Run Time System" ("Application:Kind")) -> (x = y?=w209:bool)
        n89 = Or(x=w203, y=w209) -> (x .or. y?=w207:bool)
        n90 = Bundle By Name(cluster=w208, "Core.Current VI Reference"=w206, "Core.Close Panel on Exit?"=w207) -> (w213:T11)
        n91 = call <vilib>:"Add State(s) to Queue__jki_lib_state_machine.vi"("State(s) in (\"\")"=w215) -> ("States Out"=w214:string)  [unwired: 14 in]
      }
      frame "Error Handler" {
        # "Unhandled Error -- Display it"
        # "Handle any errors here.\nYou can also output any states to clean-up after errors occur"
        # "Clear error"
        n92 = call <vilib>:"General Error Handler.vi"("error in (no error)"=w219) -> ()  [unwired: 10 in, 5 out]
        n93 = call <vilib>:"Add State(s) to Queue__jki_lib_state_machine.vi"("State(s) in Front (\"\")"="/* Post Error States", "State(s) in (\"\")"=w223) -> ("States Out"=w222:string)  [unwired: 13 in]
      }
      frame "Process Sync" {
        # "Wait on rendezvous\nCalled to synchronize with external process"
        n94 = Unbundle By Name(w227) -> ("rendezvous"=w229:T12)
        n95 = call <vilib>:"Wait at Rendezvous.vi"("error in (no error)"=w226, "ms timeout (-1)"=500, "rendezvous"=w229) -> ("error out"=w225:errorcluster)  [unwired: 2 in, 2 out]
        n96 = call <vilib>:"Add State(s) to Queue__jki_lib_state_machine.vi"("State(s) in (\"\")"=w232) -> ("States Out"=w231:string)  [unwired: 14 in]
      }
      frame "Exit" {
        # "Do not put any code in this frame.\n(No errors that occur here will be handled.)"
        n97 = call <vilib>:"Add State(s) to Queue__jki_lib_state_machine.vi"("State(s) in (\"\")"=w239) -> ("States Out"=w238:string)  [unwired: 14 in]
      }
      frame "---------- Data ----------" {
        # "Do not put any code in this frame.\n(It is a separator no-op. You can make a copy of this frame to create a new Data frame)"
        n98 = call <vilib>:"Add State(s) to Queue__jki_lib_state_machine.vi"("State(s) in (\"\")"=w245) -> ("States Out"=w244:string)  [unwired: 14 in]
      }
      frame "Data: Initialize" {
        w246 = T10 {"Font Name"="Consolas", "Size"=14, "Bold"=FALSE, "Italic"=FALSE, "Underline"=FALSE, "Strikeout"=FALSE, "Color"=7171459}  # Font
        w247 = T7[] []  # Suggestions
        w249 = -1  # T
        w253 = T9 {"Query"="", "Keywords"=[], "Position"={"Left"=0, "Top"=0}}  # Update Data
        w256 = T13 {"Current VI Reference"=refnum, "Close Panel on Exit?"=FALSE}  # Core
        # "Initialize the shift-register data, here.\n(data names are defined by what you wire into the bundle function)"
        n99 = control-ref of="List"() -> (w252:refnum<vi>)
        n100 = control-ref of="Cover"() -> (w250:refnum<vi>)
        n101 = control-ref of="Text"() -> (w251:refnum<vi>)
        n102 = Bundle("Core"=w256, "Text"=w251, "List"=w252, "Cover"=w250, "Update Data"=w253, "Suggestions"=w247, "Font"=w246, "T"=w249) -> (w257:T11)  [unwired: 1 in]
        n103 = call <vilib>:"Add State(s) to Queue__jki_lib_state_machine.vi"("State(s) in (\"\")"=w259) -> ("States Out"=w258:string)  [unwired: 14 in]
      }
      frame "Data: Register Events" {
        # "Register for dynamic events\nUser events and UI events"
        n104 = Unbundle By Name(w261) -> ("User Events"=w260:T14)
        n105 = register-events(error in=w263, w260) -> (reference out=w264:refnum<event-registration>, error out=w262:errorcluster)  [unwired: 1 in]
        n106 = call <vilib>:"Add State(s) to Queue__jki_lib_state_machine.vi"("State(s) in (\"\")"=w267) -> ("States Out"=w266:string)  [unwired: 14 in]
      }
      frame "Data: Send Suggestion" {
        # "Send selected suggestion\nCan be received by external event structures that listen for Suggestion Box public events"
        n107 = Unbundle By Name(w271) -> ("List"=w276:refnum<vi>)
        n108 = property class="LstBox (strict)"(reference=w276) -> ("Item Names"=w275:string[], "Value"=w274:i32)  [unwired: 1 in, 2 out]
        n109 = Index Array(array=w275, index=w274) -> (element=w270:string)
        n110 = call "Send Selected Suggestion Event.vi"("Suggestion Box in"=w273, "Suggestion"=w270, "error in (no error)"=w269) -> ("Suggestion Box out"=w272:refnum<class "Suggestion Box.lvclass">, "error out"=w268:errorcluster)  [unwired: 11 in]
        n111 = call <vilib>:"Add State(s) to Queue__jki_lib_state_machine.vi"("State(s) in (\"\")"=w279) -> ("States Out"=w278:string)  [unwired: 14 in]
      }
      frame "Data: Cancel Suggestion" {
        # "Send empty suggestion to cancel\nCan be received by external event structures that listen for Suggestion Box public events"
        n112 = Bundle By Name(cluster=w288, "Update Data.Keywords"=string[] []) -> (w281:T11)
        n113 = call "Send Selected Suggestion Event.vi"("Suggestion Box in"=w286, "Suggestion"="", "error in (no error)"=w284) -> ("Suggestion Box out"=w285:refnum<class "Suggestion Box.lvclass">, "error out"=w283:errorcluster)  [unwired: 11 in]
        n114 = call <vilib>:"Add State(s) to Queue__jki_lib_state_machine.vi"("State(s) in (\"\")"=w290) -> ("States Out"=w289:string)  [unwired: 14 in]
      }
      frame "Data: Set Timeout" {
        # "Set the timeout value\nArgument is integer value in milliseconds"
        n115 = Decimal String To Number(string=w291) -> (number=w292:i32)  [unwired: 2 in, 1 out]
        n116 = Bundle By Name(cluster=w296, "T"=w292) -> (w293:T11)
        n117 = call <vilib>:"Add State(s) to Queue__jki_lib_state_machine.vi"("State(s) in (\"\")"=w299) -> ("States Out"=w298:string)  [unwired: 14 in]
      }
      frame "Data: Cleanup" {
        # "Cleanup any data and references, here.\n(this is called automatically, by the Macro: Exit)"
        n118 = Unregister For Events(event registration refnum=w303, error in=w300) -> (error out=w304:errorcluster)
        n119 = Unbundle By Name(w301) -> ("Core.Current VI Reference"=w306:refnum<vi>)
        n120 = Close Reference(reference=w306, error in (no error)=w304) -> (error out=w302:errorcluster)
        n121 = call <vilib>:"Add State(s) to Queue__jki_lib_state_machine.vi"("State(s) in (\"\")"=w308) -> ("States Out"=w307:string)  [unwired: 14 in]
      }
      frame "---------- UI ----------" {
        # "Do not put any code in this frame.\n(It is a separator no-op. You can make a copy of this frame to create a new UI frame)"
        n122 = call <vilib>:"Add State(s) to Queue__jki_lib_state_machine.vi"("State(s) in (\"\")"=w314) -> ("States Out"=w313:string)  [unwired: 14 in]
      }
      frame "UI: Initialize" {
        w329 = 0 ("Value")
        # "/* Listbox is only present for the visual row highlighting -- text is not visible.\nString is overlayed on listbox, and has visible text. */"
        # "Initialize the User Interface, here.\n(this is called automatically, by the Macro: Init)"
        n123 = Unbundle By Name(w319) -> ("Font"=w317:T10)
        n124 = Unbundle By Name(w317) -> ("Size"=w316:u16, "Font Name"=w315:string)
        n125 = Unbundle By Name(w319) -> ("List"=w331:refnum<vi>)
        n126 = Unbundle By Name(w319) -> ("Text"=w324:refnum<vi>)
        n127 = Decrement(x=w316) -> (x-1=w323:u16)
        n128 = property class="LstBox (strict)"(reference=w331, "Item Names"=string[] [], "Active Row"=-2 ("Active Row:Active Row Number"), "Cell Height"=w323, "CellFontSize"=w316, "CellFontName"=w315, "Justify"=enum16{"Left", "Center", "Right"}."Left" ("Active Row:Cell Justification"), "CellFontColor"=u32 16448250, "Top Row"=w329, "Value"=w329) -> ()  [unwired: 1 in, 2 out]
        n129 = property class="Str"(reference=w324, "Text.Selection Start"=u32 0 ("Text.Selection:Start"), "Text.Selection End"=-1 ("Active Row:Active Row Number"), "Value"="", "Text.Font"=w317) -> ()  [unwired: 1 in, 2 out]
        n130 = call <vilib>:"Add State(s) to Queue__jki_lib_state_machine.vi"("State(s) in (\"\")"=w334) -> ("States Out"=w333:string)  [unwired: 14 in]
      }
      frame "UI: Cursor Set" {
        # "Argument"
        # "Set and Unset Cursor Busy.\n(Usage: \"UI: Cursor Set >> Busy|Idle\")"
        n131 = case shown="\"Idle\", Default" w337 {
          tunnel: w339 -> [w344 w346]
          tunnel: [w343 w345] -> w338
          frame "Idle", Default {
            n132 = call <vilib>:"Unset Busy.vi"("error in (no error)"=w344) -> ("error out"=w343:errorcluster)  [unwired: 10 in]
          }
          frame "Busy" {
            n133 = call <vilib>:"Set Busy.vi"("error in (no error)"=w346) -> ("error out"=w345:errorcluster)  [unwired: 9 in, 1 out]
          }
        }
        n134 = call <vilib>:"Add State(s) to Queue__jki_lib_state_machine.vi"("State(s) in (\"\")"=w342) -> ("States Out"=w341:string)  [unwired: 14 in]
      }
      frame "UI: Front Panel State" {
        # "Argument"
        # "Set Front Panel Open or Closed\n(Usage: \"UI: Front Panel State >> Open|Close\")"
        n135 = Unbundle By Name(w351) -> ("Core.Current VI Reference"=w350:refnum<vi>)
        n136 = case shown="\"Open\", \"Standard\", Default" w349 {
          tunnel: w353 -> [w361 w376 w387 w400 w413]
          tunnel: [w363 w377 w389 w402 w415] -> w352
          tunnel: w350 -> [w362 w374 w388 w401 w414]
          frame "Open", "Standard", Default {
            w356 = T1."Standard" ("State")
            n137 = property class="VI"(reference=w362, error in=w361) -> (reference out=w359:refnum<vi>, error out=w360:errorcluster, "FP.State"=w358:T1)
            n138 = Not Equal?(x=w358, y=w356) -> (x != y?=w357:bool)
            n139 = case shown="True" w357 {
              tunnel: [w367 w369] -> w363
              tunnel: w360 -> [w366 w369]
              tunnel: w359 -> [w365 _]
              tunnel: w356 -> [w364 _]
              frame True {
                n140 = invoke class="VI" method="FP.Open"(reference=w365, error in=w366, "Activate"=FALSE, "State"=w364) -> (error out=w367:errorcluster)  [unwired: 1 in, 4 out]
              }
              frame False {
              }
            }
          }
          frame "Close", "Closed" {
            n141 = property class="VI"(reference=w374, error in=w376) -> (reference out=w373:refnum<vi>, error out=w375:errorcluster, "FP.State"=w371:T1)
            n142 = Not Equal?(x=w371, y=T1."Closed" ("Front Panel Window:State")) -> (x != y?=w370:bool)
            n143 = case shown="True" w370 {
              tunnel: [w378 w381] -> w377
              tunnel: w375 -> [w378 w380]
              tunnel: w373 -> [_ w379]
              frame False {
              }
              frame True {
                n144 = invoke class="VI" method="FP.Close"(reference=w379, error in=w380) -> (error out=w381:errorcluster)  [unwired: 1 in, 2 out]
              }
            }
          }
          frame "Hidden", "Hide" {
            w382 = T1."Hidden" ("State")
            n145 = property class="VI"(reference=w388, error in=w387) -> (reference out=w385:refnum<vi>, error out=w386:errorcluster, "FP.State"=w384:T1)
            n146 = Not Equal?(x=w384, y=w382) -> (x != y?=w383:bool)
            n147 = case shown="True" w383 {
              tunnel: [w393 w394] -> w389
              tunnel: w386 -> [w392 w394]
              tunnel: w385 -> [w391 _]
              tunnel: w382 -> [w390 _]
              frame True {
                n148 = invoke class="VI" method="FP.Open"(reference=w391, error in=w392, "State"=w390) -> (error out=w393:errorcluster)  [unwired: 2 in, 4 out]
              }
              frame False {
              }
            }
          }
          frame "Minimize", "Minimized" {
            w395 = T1."Minimized" ("State")
            n149 = property class="VI"(reference=w401, error in=w400) -> (reference out=w398:refnum<vi>, error out=w399:errorcluster, "FP.State"=w397:T1)
            n150 = Not Equal?(x=w397, y=w395) -> (x != y?=w396:bool)
            n151 = case shown="True" w396 {
              tunnel: [w406 w407] -> w402
              tunnel: w399 -> [w405 w407]
              tunnel: w398 -> [w404 _]
              tunnel: w395 -> [w403 _]
              frame True {
                n152 = invoke class="VI" method="FP.Open"(reference=w404, error in=w405, "State"=w403) -> (error out=w406:errorcluster)  [unwired: 2 in, 4 out]
              }
              frame False {
              }
            }
          }
          frame "Maximize", "Maximized" {
            w408 = T1."Maximized" ("State")
            n153 = property class="VI"(reference=w414, error in=w413) -> (reference out=w411:refnum<vi>, error out=w412:errorcluster, "FP.State"=w410:T1)
            n154 = Not Equal?(x=w410, y=w408) -> (x != y?=w409:bool)
            n155 = case shown="True" w409 {
              tunnel: [w419 w420] -> w415
              tunnel: w412 -> [w418 w420]
              tunnel: w411 -> [w417 _]
              tunnel: w408 -> [w416 _]
              frame True {
                n156 = invoke class="VI" method="FP.Open"(reference=w417, error in=w418, "State"=w416) -> (error out=w419:errorcluster)  [unwired: 2 in, 4 out]
              }
              frame False {
              }
            }
          }
        }
        n157 = call <vilib>:"Add State(s) to Queue__jki_lib_state_machine.vi"("State(s) in (\"\")"=w355) -> ("States Out"=w354:string)  [unwired: 14 in]
      }
      frame "UI: Defer Updates" {
        # "Defer panel updates\n(Usage: \"UI: Defer Updates >> True|False\")"
        n158 = Unbundle By Name(w429) -> ("Core.Current VI Reference"=w421:refnum<vi>)
        n159 = case shown="\"True\"" w430 {
          tunnel: [FALSE TRUE] -> w422
          frame "False", Default {
          }
          frame "True" {
          }
        }
        n160 = property class="VI"(reference=w421, error in=w423) -> (error out=w427:errorcluster, "Panel"=w428:refnum<vi>)  [unwired: 1 out]
        n161 = property class="Pnl"(reference=w428, error in=w427, "DeferPanUpdts"=w422) -> (reference out=w425:refnum<vi>, error out=w426:errorcluster)
        n162 = Close Reference(reference=w425, error in (no error)=w426) -> (error out=w424:errorcluster)
        n163 = call <vilib>:"Add State(s) to Queue__jki_lib_state_machine.vi"("State(s) in (\"\")"=w434) -> ("States Out"=w433:string)  [unwired: 14 in]
      }
      frame "UI: Populate" {
        # "Fill in the listbox and the backing text\nListbox items are not visible. Emphasize the string characters that match the query"
        n164 = Unbundle By Name(w442) -> ("Suggestions"=w439:T7[])
        n165 = Unbundle By Name(w442) -> ("List"=w441:refnum<vi>)
        n166 = Unbundle By Name(w442) -> ("Text"=w443:refnum<vi>)
        n167 = Empty Array?(array=w439) -> (empty?=w440:bool)
        n168 = case shown="False" w440 {
          tunnel: w439 -> [w450 _]
          tunnel: w443 -> [w454 _]
          tunnel: w441 -> [w452 _]
          tunnel: [w449 _] -> w437
          frame False {
            n169 = for {
              tunnel: w450 -> [w461] mode=indexing
              tunnel: [w459] -> w449 mode=indexing
              shift-right: [w460] -> w451
              shift-left: "" -> [w457]
              n170 = Unbundle By Name(w461) -> ("Source"=w459:string)
              n171 = Empty String/Path?(string/path=w457) -> (empty?=w458:bool)
              n172 = Select(t=w457, s=w458, f="\n") -> (s? t:f=w455:string)
              n173 = Concatenate Strings(w457, w455, w459) -> (w460:string)
            }
            n174 = property class="LstBox (strict)"(reference=w452, "Item Names"=w449) -> ()  [unwired: 1 in, 2 out]
            n175 = local write "Text"(w451) -> ()
            n176 = call "Emphasize Query.vi"("String Ref in"=w454, "Suggestions"=w450, "Lines"=w449) -> ()  [unwired: 13 in]
          }
          frame True {
          }
        }
        n177 = Bundle By Name(cluster=w442, "Update Data.Keywords"=w437) -> (w438:T11)
        n178 = call <vilib>:"Add State(s) to Queue__jki_lib_state_machine.vi"("State(s) in (\"\")"=w448) -> ("States Out"=w447:string)  [unwired: 14 in]
      }
      frame "UI: Size" {
        w470 = u32 18  # Scrollbar Width
        # "Set the panel size\nAutoscale the listbox width via text, and height via number of items, then set the panel bounds and refit listbox"
        n179 = Unbundle By Name(w462) -> ("Core.Current VI Reference"=w484:refnum<vi>)
        n180 = Unbundle By Name(w462) -> ("Update Data.Position.Left"=w478:i32, "Update Data.Position.Top"=w477:i32)
        n181 = Unbundle By Name(w462) -> ("List"=w468:refnum<vi>)
        n182 = Unbundle By Name(w462) -> ("Text"=w474:refnum<vi>)
        n183 = Unbundle By Name(w462) -> ("Cover"=w469:refnum<vi>)
        n184 = call "Get Auto-Sized Listbox Dimensions.vi"("Listbox Ref"=w468) -> ("Listbox Ref out"=w465:refnum<vi>, "Width"=w464:u32, "Height"=w463:u32)  [unwired: 11 in, 1 out]
        n185 = Add(x=w464, y=w478) -> (x+y=w479:u32)
        n186 = property class="VI"(reference=w484) -> (reference out=w482:refnum<vi>, "Front Panel.PanelBounds"=w481:T4)  [unwired: 1 in, 1 out]
        n187 = Add(x=w463, y=w477) -> (x+y=w480:u32)
        n188 = property class="Pict"(reference=w469) -> (reference out=w472:refnum<vi>, "Draw Area Size"=w467:T15)  [unwired: 1 in, 1 out]
        n189 = Bundle By Name(cluster=w481, "Right"=w479, "Bottom"=w480, "Left"=w478, "Top"=w477) -> (w483:T4)
        n190 = property class="VI"(reference=w482, "Front Panel.PanelBounds"=w483) -> (error out=w473:errorcluster)  [unwired: 1 in, 1 out]
        n191 = Subtract(x=w464, y=w470) -> (x-y=w466:u32)
        n192 = property class="LstBox (strict)"(reference=w465, "Width"=w464, "Height"=w463) -> ()  [unwired: 1 in, 2 out]
        n193 = property class="Str"(reference=w474, "Height"=w463, "Width"=w466) -> ()  [unwired: 1 in, 2 out]
        n194 = Bundle By Name(cluster=w467, "Width"=w466, "Height"=w463) -> (w471:T15)
        n195 = call <vilib>:"Clear Errors.vi"("error in (no error)"=w473) -> ()  [unwired: 5 in, 2 out]
        n196 = property class="Pict"(reference=w472, "Draw Area Size"=w471) -> ()  [unwired: 1 in, 2 out]
        n197 = call <vilib>:"Add State(s) to Queue__jki_lib_state_machine.vi"("State(s) in (\"\")"=w487) -> ("States Out"=w486:string)  [unwired: 14 in]
      }
      frame "UI: Navigate" {
        # "Do not put any code in this frame.\n(It is a separator no-op. You can make a copy of this frame to create a new UI frame)"
        n198 = Decimal String To Number(string=w490) -> (number=w489:i32)  [unwired: 2 in, 1 out]
        n199 = Unbundle By Name(w492) -> ("List"=w491:refnum<vi>)
        n200 = property class="LstBox (strict)"(reference=w491, "Value"=w489) -> ("Top Row"=w494:i32, "Number of Rows"=w500:u32)  [unwired: 1 in, 2 out]
        n201 = To Long Integer(number=w500) -> (32bit integer=w499:i32)
        n202 = Add(x=w494, y=w499) -> (x+y=w496:i32)
        n203 = Less Or Equal?(x=w496, y=w489) -> (x <= y?=w495:bool)
        n204 = case shown="False" w495 {
          tunnel: w494 -> [w508 _]
          tunnel: [w509 1 ("Top Row")] -> w493
          tunnel: w489 -> [w507 _]
          frame False {
            n205 = Greater?(x=w508, y=w507) -> (0:w506:bool)
            n206 = case shown="False" w506 {
              tunnel: [0 ("Top Row") -1 ("Top Row")] -> w509
              frame False {
              }
              frame True {
              }
            }
          }
          frame True {
          }
        }
        n207 = Number To Decimal String(number=w493) -> (decimal integer string=w497:string)  [unwired: 1 in]
        n208 = call <vilib>:"Build State String with Arguments__jki_lib_state_machine.vi"("Arguments (\"\")"=w497, "State"="UI: Scroll") -> ("State with Arguments"=w488:string)  [unwired: 4 in]
        n209 = call <vilib>:"Add State(s) to Queue__jki_lib_state_machine.vi"("State(s) in Front (\"\")"=w488, "State(s) in (\"\")"=w505) -> ("States Out"=w504:string)  [unwired: 13 in]
      }
      frame "UI: Scroll" {
        # "Scroll the Suggestion Box\nNeed to adjust the text and listbox"
        n210 = Decimal String To Number(string=w514) -> (number=w513:i32)  [unwired: 2 in, 1 out]
        n211 = Unbundle By Name(w515) -> ("Text"=w522:refnum<vi>)
        n212 = Unbundle By Name(w515) -> ("List"=w527:refnum<vi>)
        n213 = property class="LstBox (strict)"(reference=w527) -> (reference out=w523:refnum<vi>, "Item Names"=w524:string[], "Number of Rows"=w520:u32, "Top Row"=w516:i32)  [unwired: 1 in, 1 out]
        n214 = To Long Integer(number=w520) -> (32bit integer=w517:i32)
        n215 = Array Size(array=w524) -> (size(s)=w521:i32)
        n216 = Subtract(x=w521, y=w517) -> (x-y=w519:i32)
        n217 = Add(x=w516, y=w513) -> (x+y=w526:i32)
        n218 = In Range and Coerce(upper limit=w519, x=w526, lower limit=0) -> (coerced(x)=w518:i32)  [unwired: 1 out]
        n219 = property class="Str"(reference=w522, "Text.Scroll Position"=w518) -> ()  [unwired: 1 in, 2 out]
        n220 = property class="LstBox (strict)"(reference=w523, "Top Row"=w518) -> ()  [unwired: 1 in, 2 out]
        n221 = call <vilib>:"Add State(s) to Queue__jki_lib_state_machine.vi"("State(s) in (\"\")"=w532) -> ("States Out"=w531:string)  [unwired: 14 in]
      }
      frame "UI: Cleanup" {
        # "Initialize the User Interface, here.\n(this is called automatically, by the Macro: Init)"
        n222 = Unbundle By Name(w540) -> ("Text"=w534:refnum<vi>, "List"=w539:refnum<vi>)
        n223 = property class="Str"(reference=w534, "Value"="") -> ()  [unwired: 1 in, 2 out]
        n224 = property class="LstBox (strict)"(reference=w539, "Item Names"=string[] [], "Scrollbar Visible"=FALSE ("Visible Items:Vertical Scrollbar Visible")) -> ()  [unwired: 1 in, 2 out]
        n225 = call <vilib>:"Add State(s) to Queue__jki_lib_state_machine.vi"("State(s) in (\"\")"=w543) -> ("States Out"=w542:string)  [unwired: 14 in]
      }
      frame "---------- Macro ----------" {
        # "Do not put any code in this frame.\n(It is a separator no-op. You can make a copy of this frame to create a new Macro frame)"
        n226 = call <vilib>:"Add State(s) to Queue__jki_lib_state_machine.vi"("State(s) in (\"\")"=w549) -> ("States Out"=w548:string)  [unwired: 14 in]
      }
      frame "Macro: Initialize" {
        # "Initialization Macro\n(This is called once, when the VI starts)"
        n227 = call <vilib>:"Add State(s) to Queue__jki_lib_state_machine.vi"("State(s) in Front (\"\")"="Data: Initialize\nInitialize Core Data\nUI: Initialize\nData: Register Events\nProcess Sync\n//UI: Front Panel State >> Open", "State(s) in (\"\")"=w556) -> ("States Out"=w555:string)  [unwired: 13 in]
      }
      frame "Macro: Display" {
        # "Display the suggestion box\nPopulate, size, and open the panel, and then turn on timeout events"
        n228 = call <vilib>:"Add State(s) to Queue__jki_lib_state_machine.vi"("State(s) in Front (\"\")"="UI: Defer Updates >> True\nUI: Initialize\nUI: Populate\nUI: Size\nUI: Front Panel State >> Open\nUI: Defer Updates >> False\nData: Set Timeout >> 50", "State(s) in (\"\")"=w563) -> ("States Out"=w562:string)  [unwired: 13 in]
      }
      frame "Macro: Navigate" {
        # "Do not put any code in this frame.\n(It is a separator no-op. You can make a copy of this frame to create a new Macro frame)"
        n229 = call <vilib>:"Build State String with Arguments__JKI_lib_State_Machine.vi"("Arguments (\"\")"=w568, "State"="UI: Navigate") -> ("State with Arguments"=w566:string)  [unwired: 4 in]
        n230 = call <vilib>:"Add State(s) to Queue__jki_lib_state_machine.vi"("State(s) in Front (\"\")"="UI: Defer Updates >> True", "State(s) in (\"\")"=w566, "State(s) at Back (\"\")"="UI: Defer Updates >> False") -> ("States Out"=w564:string)  [unwired: 12 in]
        n231 = call <vilib>:"Add State(s) to Queue__jki_lib_state_machine.vi"("State(s) in Front (\"\")"=w564, "State(s) in (\"\")"=w575) -> ("States Out"=w574:string)  [unwired: 13 in]
      }
      frame "Macro: Accept" {
        # "Accept the selected suggestion\nStop the timeout event, send the selected item out to listeners, and close the panel"
        n232 = call <vilib>:"Add State(s) to Queue__jki_lib_state_machine.vi"("State(s) in Front (\"\")"="Data: Set Timeout >> -1\nData: Send Suggestion\nUI: Front Panel State >> Hide", "State(s) in (\"\")"=w582) -> ("States Out"=w581:string)  [unwired: 13 in]
      }
      frame "Macro: Cancel" {
        # "Cancel the suggestion selection\nStop the timeout event and close the panel"
        n233 = call <vilib>:"Add State(s) to Queue__jki_lib_state_machine.vi"("State(s) in Front (\"\")"="Data: Set Timeout >> -1\nData: Cancel Suggestion\nUI: Front Panel State >> Hide", "State(s) in (\"\")"=w589) -> ("States Out"=w588:string)  [unwired: 13 in]
      }
      frame "Macro: Exit" {
        # "Exit Macro\n(This is called once, when the VI exits)"
        n234 = case shown="\"Sync\"" w593 {
          tunnel: [_ "Process Sync"] -> w594
          frame Default {
          }
          frame "Sync" {
          }
        }
        n235 = call <vilib>:"Add State(s) to Queue__jki_lib_state_machine.vi"("State(s) in Front (\"\")"="UI: Cleanup\nData: Cleanup", "State(s) in (\"\")"=w594, "State(s) at Back (\"\")"="Exit") -> ("States Out"=w595:string)  [unwired: 12 in]
        n236 = call <vilib>:"Add State(s) to Queue__jki_lib_state_machine.vi"("State(s) in (\"\")"="UI: Front Panel State >> Close", "State(s) at Back (\"\")"=w595) -> ("States Out"=w591:string)  [unwired: 13 in]
        n237 = call <vilib>:"Add State(s) to Queue__jki_lib_state_machine.vi"("State(s) in Front (\"\")"=w591, "State(s) in (\"\")"=w602) -> ("States Out"=w601:string)  [unwired: 13 in]
      }
    }
  }
